vi "GLB_Timing.vi"() -> ()   [LabVIEW 2014, in "PLS Digital Control.lvlib"]
uses:
  PLS Digital Control.lvlib
panel:
  in  "L4":cluster{"Tcold":dbl, "Twarm":dbl}={"Tcold"=5.0, "Twarm"=5.0} {"Twarm" min=5.0 max=1000.0 step=0.1 format="%d s"; "Tcold" min=5.0 max=1000.0 step=0.1 format="%d s"}
  in  "L1":cluster{"Topen":dbl, "Tclose":dbl}={"Topen"=5.0, "Tclose"=5.0} {"Tclose" min=5.0 max=1000.0 step=0.1 format="%d s"; "Topen" min=5.0 max=1000.0 step=0.1 format="%d s"}
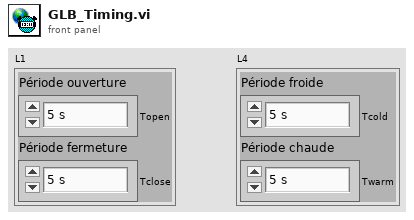
[diagram p1: front panel]
diagram:
